vi "Parse frame container to string array.vi"(1 "Frame":T1 {"Data" format="%.0x"}) -> (0 "String array":string[](array[string]))   [LabVIEW 2021, in "uCanDriver.lvlib" / "uCAN.lvclass"]
uses:
  uCAN.lvclass
  typedefs/frame.ctl
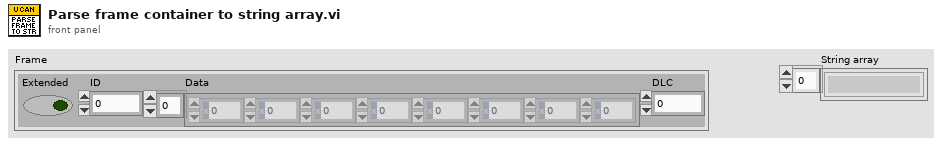
[diagram p1: front panel]
types:
  T1 = typedef "uCanDriver.lvlib/uCAN.lvclass/frame.ctl" = cluster{"Extended":bool, "ID":u32, "Data":u8[], "DLC":u8}
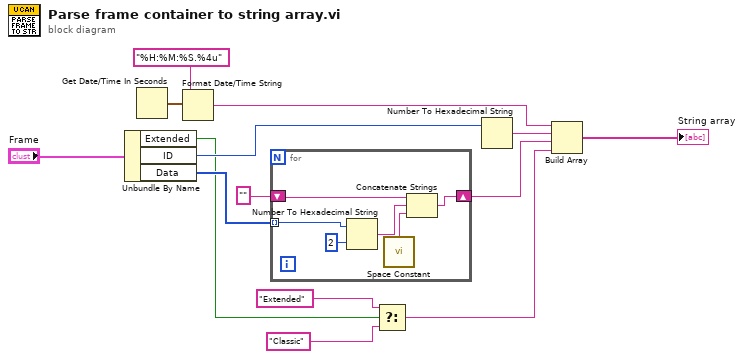
[diagram p0: block diagram]
diagram:
  n1 = Unbundle By Name("Frame") -> ("Extended"=w6:bool, "ID"=w11:u32, "Data"=w8:u8[])
  n2 = Get Date/Time In Seconds() -> (seconds since 1Jan1904=w14:timestamp)
  n3 = Format Date/Time String(time format string (%c)="%H:%M:%S.%4u", seconds (now)=w14) -> (date/time string=w12:string)  [unwired: 1 in]
  n4 = for {
    shift-right: [w16] -> w7
    shift-left: "" ("time format string (%c)") -> [w20]
    tunnel: w8 -> [w19] mode=indexing
    n5 = Number To Hexadecimal String(1:i16 2 ("width (-)"), 2:w19) -> (0:w18:string)
    n6 = call <vilib>:"Space Constant.vi"() -> ("String"=w17:string)
    n7 = Concatenate Strings(w20, w18, w17) -> (w16:string)
  }
  n8 = Select(t="Extended" ("time format string (%c)"), s=w6, f="Classic" ("time format string (%c)")) -> (s? t:f=w5:string)
  n9 = Number To Hexadecimal String(2:w11) -> (0:w10:string)  [unwired: 1 in]
  n10 = Build Array(w12, w10, w7, w5) -> (→"String array":string[])
